vi "Read I-V parameters.vi"(8 "error in (no error)":errorcluster, 11 "RP I-V Driver in":refnum<class "RP I-V Driver.lvclass">) -> (0 "error out":errorcluster, 2 "I-V parameters":T1={"Start magnitude"=0.01, "Magnitude increment"=0.001, "End magnitude"=8.0, "Baseline length"=0, "Ramp length"=0, "Top  length"=0, "Threshold "=1e-05, "Processing delay"=255, "Valhalla range"=0.001, "Interpolation"=64} {"Valhalla range" format="%#_6pA"; "Processing delay" format="%dpts"; "Threshold" format="%#_6pV"; "Top  length" format="%dpts"; "Ramp length" format="%dpts"; "Baseline length" format="%dpts"; "End magnitude" format="%#_6pA"; "Magnitude increment" format="%#_6pA"; "Start magnitude" format="%#_6pA"}, 3 "RP I-V Driver out":refnum<class "RP I-V Driver.lvclass">)   [LabVIEW 2016, in "RP I-V Driver.lvclass"]
uses:
  RP I-V Driver.lvclass
  Waform generation/I-V parameters.ctl
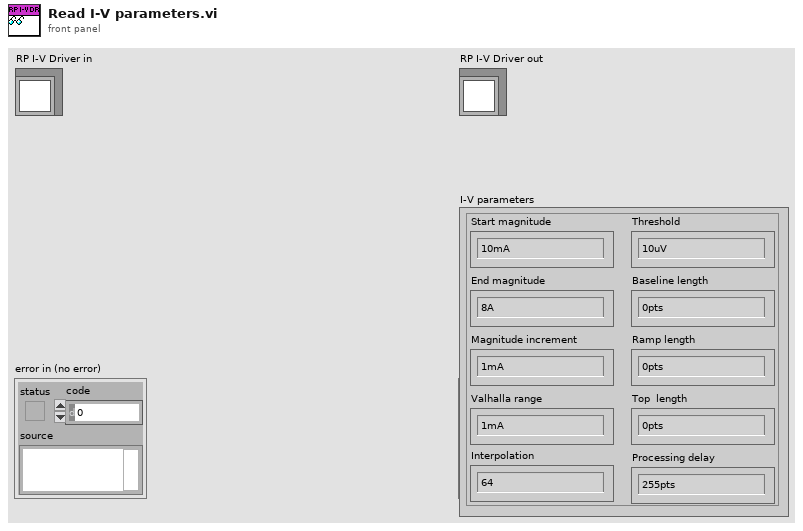
[diagram p1: front panel]
types:
  T1 = typedef "I-V parameters.ctl" = cluster{"Start magnitude":dbl, "Magnitude increment":dbl, "End magnitude":dbl, "Baseline length":i32, "Ramp length":i32, "Top  length":i32, "Threshold ":dbl, "Processing delay":u16, "Valhalla range":dbl, "Interpolation":i32}
  T2 = typedef "RP I-V Configuration.ctl" = cluster{"I-V parameters":T1, "Ranges":dbl[], "Pre-trigger duration":dbl, "Post-trigger duration":dbl, "Output delay":dbl}
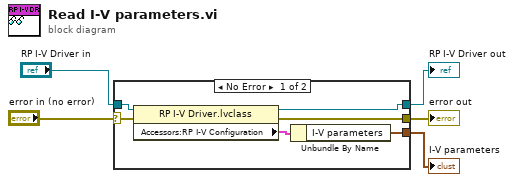
[diagram p0: block diagram]
diagram:
  n1 = case shown="No Error" "error in (no error)" {
    selector: "error in (no error)" -> [w11 w12]
    tunnel: [w9 w12] -> w4
    tunnel: [w7 w13] -> w2
    tunnel: "RP I-V Driver in" -> [w8 w13]
    tunnel: [w10 _] -> w1
    frame No Error {
      n2 = property class="RP I-V Driver.lvclass"(reference=w8, error in=w11) -> (reference out=w7:refnum<class "RP I-V Driver.lvclass">, error out=w9:errorcluster, "Accessors:RP I-V Configuration"=w6:T2)
      n3 = Unbundle By Name(w6) -> ("I-V parameters"=w10:T1)
    }
    frame Error {
    }
  }
  "error out" <- w4
  "RP I-V Driver out" <- w2
  "I-V parameters" <- w1
